vi "MessageHandler__LCR.vi"(6 "reference":T11, 7 "Data In":T3, 8 "error in (no error)":errorcluster, 9 "Action In":T4 caption="Action", 10 "Message":T1={"Command"=enum."SetPicture", "Parameter"=variant} caption="Messages", 11 "State In":T5={"Orientation"=0, "ActivePicture"={"image type"=0, "image depth"=0, "image"=[], "mask"=[], "colors"=[], "Rectangle"={"left"=0, "top"=0, "right"=0, "bottom"=0}}, "Pictures"={"Normal"={"image type"=0, "image depth"=0, "image"=[], "mask"=[], "colors"=[], "Rectangle"={"left"=0, "top"=0, "right"=0, "bottom"=0}}, "Hilite"={"image type"=0, "image depth"=0, "image"=[], "mask"=[], "colors"=[], "Rectangle"={"left"=0, "top"=0, "right"=0, "bottom"=0}}}, "Text"={"String"="", "Font"={"Font Name:"="", "Size"=0, "Strikeout?"=FALSE, "Italic?"=FALSE, "Underline?"=FALSE, "Outline?"=FALSE, "Shadow?"=FALSE, "Bold?"=FALSE}, "TextColor"=0}, "RunTimeSettings"={"Highlight"=FALSE, "ShowButton"=TRUE, "Behaviour"=enum."Switch when pressed", "React if disabled"=FALSE, "Nudge Button"=TRUE, "ShowButton on Hover"=FALSE, "Button Type"=enum."System"}, "Messages"=[], "Status"=0, "XControl Label"="", "Boolean Value"=FALSE} caption="State" {"Status" format="%.0x"}) -> (0 "error out":errorcluster, 1 "Action Out":T4 caption="Action", 2 "Remaining":i32, 3 "State Out":T5={"Orientation"=0, "ActivePicture"={"image type"=0, "image depth"=0, "image"=[], "mask"=[], "colors"=[], "Rectangle"={"left"=0, "top"=0, "right"=0, "bottom"=0}}, "Pictures"={"Normal"={"image type"=0, "image depth"=0, "image"=[], "mask"=[], "colors"=[], "Rectangle"={"left"=0, "top"=0, "right"=0, "bottom"=0}}, "Hilite"={"image type"=0, "image depth"=0, "image"=[], "mask"=[], "colors"=[], "Rectangle"={"left"=0, "top"=0, "right"=0, "bottom"=0}}}, "Text"={"String"="", "Font"={"Font Name:"="", "Size"=0, "Strikeout?"=FALSE, "Italic?"=FALSE, "Underline?"=FALSE, "Outline?"=FALSE, "Shadow?"=FALSE, "Bold?"=FALSE}, "TextColor"=0}, "RunTimeSettings"={"Highlight"=FALSE, "ShowButton"=TRUE, "Behaviour"=enum."Switch when pressed", "React if disabled"=FALSE, "Nudge Button"=TRUE, "ShowButton on Hover"=FALSE, "Button Type"=enum."System"}, "Messages"=[], "Status"=0, "XControl Label"="", "Boolean Value"=FALSE} caption="State" {"Status" format="%.0x"})   [LabVIEW 2011, in "BooleanXControl__LCR.xctl"]
uses:
  BooleanXControl__LCR.xctl
  Controls/BX.Refs__LCR.ctl
  Abilities/BX.State__LCR.ctl
  Controls/BX.Orientation__LCR.ctl
  <vilib>/picture/picture.llb/imagedata.ctl
  Controls/BX.RTSettings__LCR.ctl
  Controls/BX.Behaviour__LCR.ctl
  Controls/BX.ButtonType__LCR.ctl
  Controls/BX.Message__LCR.ctl
  Controls/BX.Commands__LCR.ctl
  <vilib>/_xctls/Action.ctl
  Abilities/BX.Data__LCR.ctl
  <vilib>/_xctls/XControlSupport.lvlib
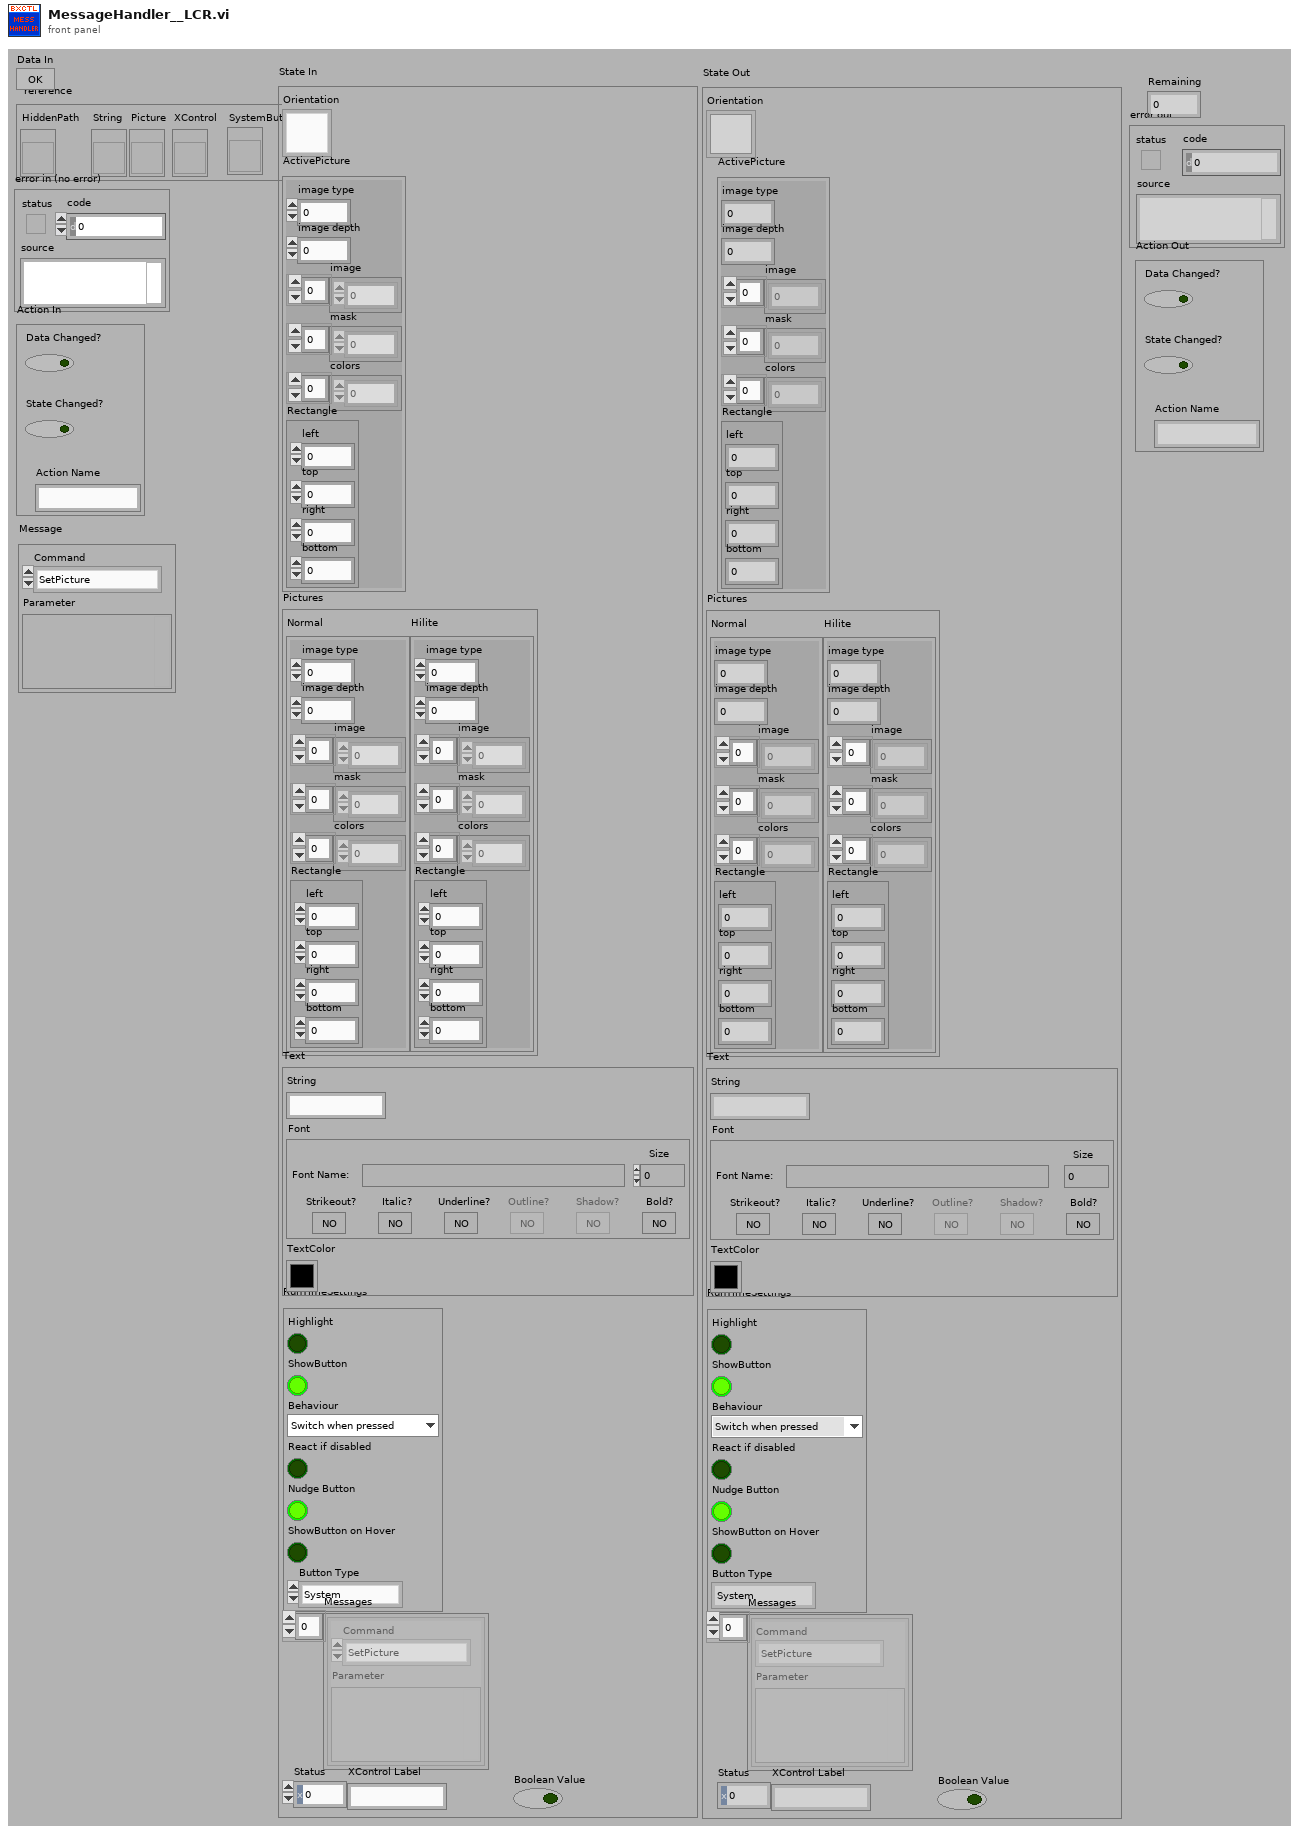
[diagram p1: front panel]
types:
  T1 = typedef "BooleanXControl__LCR.xctl/BX.Message__LCR.ctl" = cluster{"Command":T2, "Parameter":variant}
  T2 = typedef "BooleanXControl__LCR.xctl/BX.Commands__LCR.ctl" = enum16{"None", "SetPicture", "SetFont", "SetText", "SetOrientation", "Redraw", "SetTextColor", "SetRTSettings", "MultipleUpdate", "RT.Button", "RT.Hilite", "RT.Behaviour", "RT.Disabled", "ShowGUI", "RT.Nudge", "RT.Hover", "RT.ButtonType"}
  T3 = typedef "BooleanXControl__LCR.xctl/BX.Data__LCR.ctl" = bool
  T4 = typedef "XControlSupport.lvlib/Action.ctl" = cluster{"Data Changed?":bool, "State Changed?":bool, "Action Name":string}
  T5 = typedef "BooleanXControl__LCR.xctl/BX.State__LCR.ctl" = cluster{"Orientation":T6, "ActivePicture":T7, "Pictures":cluster{"Normal":T7, "Hilite":T7}, "Text":cluster{"String":string, "Font":cluster{"Font Name:":string, "Size":i16, "Strikeout?":bool, "Italic?":bool, "Underline?":bool, "Outline?":bool, "Shadow?":bool, "Bold?":bool}, "TextColor":u32}, "RunTimeSettings":T8, "Messages":T1[], "Status":u16, "XControl Label":string, "Boolean Value":bool}
  T6 = typedef "BooleanXControl__LCR.xctl/BX.Orientation__LCR.ctl" = u8
  T7 = typedef "imagedata.ctl" = cluster{"image type":i32, "image depth":i32, "image":u8[], "mask":u8[], "colors":u32[], "Rectangle":cluster{"left":i16, "top":i16, "right":i16, "bottom":i16}}
  T8 = typedef "BooleanXControl__LCR.xctl/BX.RTSettings__LCR.ctl" = cluster{"Highlight":bool, "ShowButton":bool, "Behaviour":T9, "React if disabled":bool, "Nudge Button":bool, "ShowButton on Hover":bool, "Button Type":T10}
  T9 = typedef "BooleanXControl__LCR.xctl/BX.Behaviour__LCR.ctl" = enum16{"Switch when pressed", "Switch when released", "Switch until released"}
  T10 = typedef "BooleanXControl__LCR.xctl/BX.ButtonType__LCR.ctl" = enum16{"System", "Modern", "Classic", "Decoration"}
  T11 = typedef "BooleanXControl__LCR.xctl/BX.Refs__LCR.ctl" = cluster{"HiddenPath":refnum<vi>, "String":refnum<vi>, "Picture":refnum<vi>, "XControl":refnum<vi>, "SystemButton":refnum<vi>, "ModernButton":refnum<vi>, "ClassicButton":refnum<vi>, "Decor Refnum":refnum<vi>}
  T12 = cluster{"Font Name:":string, "Size":i16, "Strikeout?":bool, "Italic?":bool, "Underline?":bool, "Outline?":bool, "Shadow?":bool, "Bold?":bool}
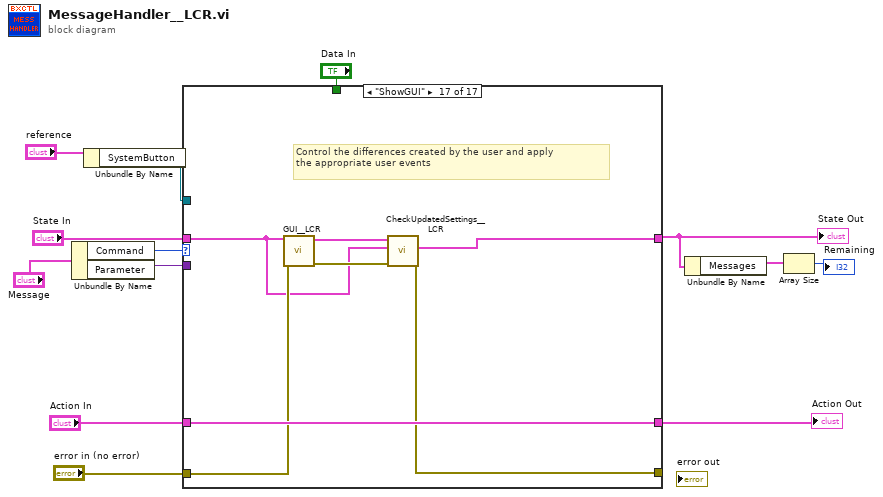
[diagram p0: block diagram]
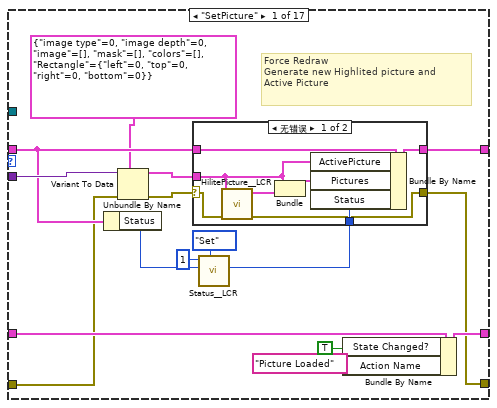
[diagram p2: hidden frame]
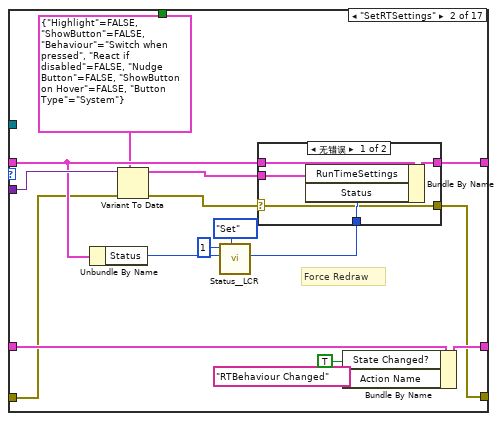
[diagram p4: hidden frame]
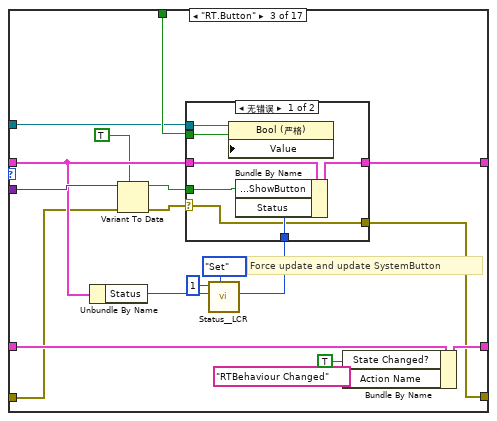
[diagram p6: hidden frame]
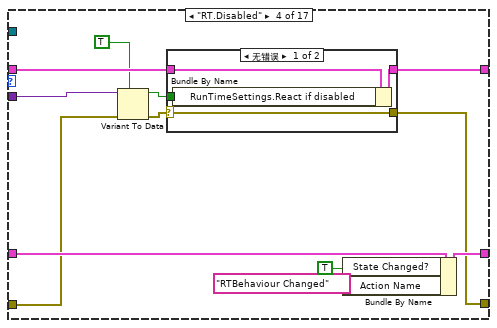
[diagram p8: hidden frame]
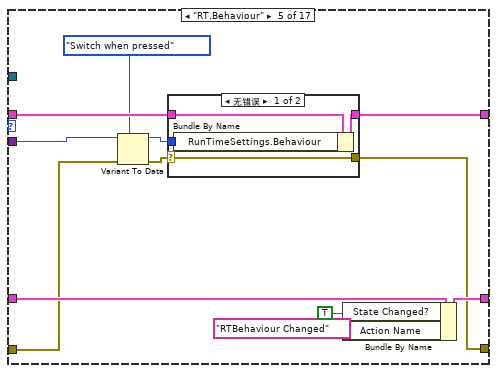
[diagram p10: hidden frame]
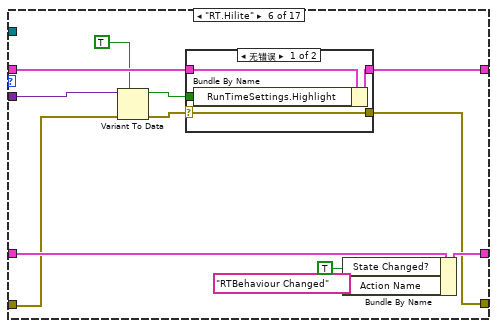
[diagram p12: hidden frame]
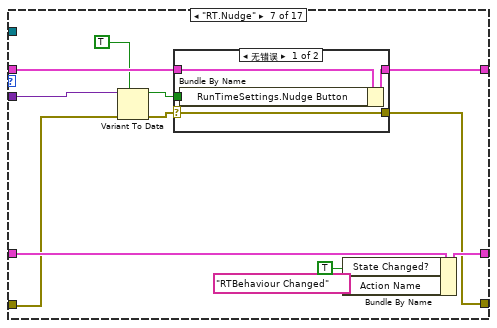
[diagram p14: hidden frame]
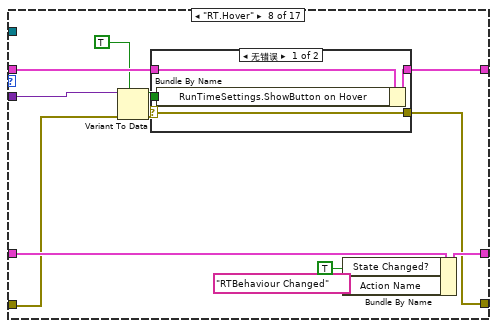
[diagram p16: hidden frame]
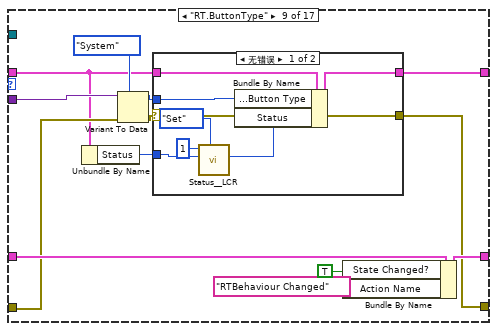
[diagram p18: hidden frame]
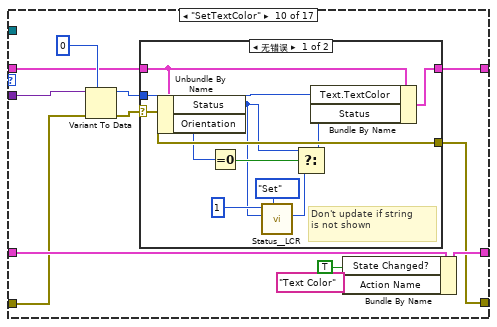
[diagram p20: hidden frame]
diagram:
  n1 = Unbundle By Name("Message") -> ("Command"=w5:T2, "Parameter"=w4:variant)
  n2 = Unbundle By Name("reference") -> ("SystemButton"=w8:refnum<vi>)
  n3 = case shown="\"ShowGUI\"" w5 {
    tunnel: w4 -> [w28 w54 w79 w100 w118 w136 w154 w172 w191 w213 w239 w264 w288 _ _ w322 _]
    tunnel: "State In" -> [w22 w48 w73 w94 w112 w130 w148 w166 w181 w206 w229 w255 w281 w309 w313 w315 w328]
    tunnel: "Action In" -> [w27 w53 w78 w99 w117 w135 w153 w171 w190 w211 w238 w263 w287 w310 w312 w323 w333]
    tunnel: [w26 w52 w77 w98 w116 w134 w152 w170 w189 w210 w237 w262 w286 w310 w312 w323 w333] -> w12
    tunnel: [w29 w55 w80 w101 w119 w137 w155 w173 w192 w214 w228 w254 w289 w308 w313 w314 w329] -> w3
    tunnel: "error in (no error)" -> [w19 w45 w70 w91 w109 w127 w145 w163 w183 w204 w233 w258 w279 w307 w311 w318 w332]
    tunnel: [w18 w44 w69 w90 w108 w126 w144 w162 w182 w203 w232 w253 w278 w307 w311 w316 w330] -> _
    tunnel: "Data In" -> [_ _ w68 _ _ _ _ _ _ _ _ _ _ _ _ _ _]
    tunnel: w8 -> [_ _ w67 _ _ _ _ _ _ _ _ _ _ _ _ _ _]
    frame "SetPicture" {
      # "Force Redraw\nGenerate new Highlited picture and\nActive Picture"
      n4 = Unbundle By Name(w22) -> ("Status"=w17:u16)
      n5 = Variant To Data(error in=w19, type=T7 {"image type"=0, "image depth"=0, "image"=[], "mask"=[], "colors"=[], "Rectangle"={"left"=0, "top"=0, "right"=0, "bottom"=0}} ("image data"), Variant=w28) -> (data=w23:T7, error out=w21:errorcluster)
      n6 = call "Status__LCR.vi"("Action (Get)"=enum16{"Get", "Set", "Reset"}."Set", "Status In"=w17, "Bit"=u16 1) -> ("Status Out"=w14:u16)  [unwired: 7 in, 1 out]
      n7 = case shown="无错误" w21 {
        selector: w21 -> [w31 w38]
        tunnel: [w37 w39] -> w29
        tunnel: w23 -> [w34 _]
        tunnel: w22 -> [w33 w39]
        tunnel: w14 -> [w32 _]
        tunnel: [w30 w38] -> w18
        frame No Error {
          n8 = call "HilitePicture__LCR.vi"("error in (no error)"=w31, "image data"=w34) -> ("error out"=w30:errorcluster, "Hilited Picture"=w36:T7)  [unwired: 8 in]
          n9 = Bundle("image data"=w34, "Hilited Picture"=w36) -> (w35:cluster{"image data":T7, "Hilited Picture":T7})  [unwired: 1 in]
          n10 = Bundle By Name(cluster=w33, "ActivePicture"=w34, "Pictures"=w35, "Status"=w32) -> (w37:T5)
        }
        frame Error {
          # "Wrong datatype"
        }
      }
      n11 = Bundle By Name(cluster=w27, "State Changed?"=TRUE ("Data Changed?"), "Action Name"="Picture Loaded") -> (w26:T4)
    }
    frame "SetRTSettings" {
      # "Force Redraw"
      n12 = Unbundle By Name(w48) -> ("Status"=w41:u16)
      n13 = Variant To Data(error in=w45, type=T8 {"Highlight"=FALSE, "ShowButton"=FALSE, "Behaviour"=enum."Switch when pressed", "React if disabled"=FALSE, "Nudge Button"=FALSE, "ShowButton on Hover"=FALSE, "Button Type"=enum."System"} ("RunTimeSettings"), Variant=w54) -> (data=w49:T8, error out=w47:errorcluster)
      n14 = call "Status__LCR.vi"("Action (Get)"=enum16{"Get", "Set", "Reset"}."Set", "Status In"=w41, "Bit"=u16 1) -> ("Status Out"=w40:u16)  [unwired: 7 in, 1 out]
      n15 = case shown="无错误" w47 {
        selector: w47 -> [w56 w61]
        tunnel: [w60 w62] -> w55
        tunnel: w49 -> [w59 _]
        tunnel: w48 -> [w58 w62]
        tunnel: w40 -> [w57 _]
        tunnel: [w56 w61] -> w44
        frame No Error {
          n16 = Bundle By Name(cluster=w58, "RunTimeSettings"=w59, "Status"=w57) -> (w60:T5)
        }
        frame Error {
          # "Wrong Datatype"
        }
      }
      n17 = Bundle By Name(cluster=w53, "State Changed?"=TRUE ("Data Changed?"), "Action Name"="RTBehaviour Changed") -> (w52:T4)
    }
    frame "RT.Button" {
      # "Force update and update SystemButton"
      n18 = Unbundle By Name(w73) -> ("Status"=w64:u16)
      n19 = Variant To Data(error in=w70, type=TRUE, Variant=w79) -> (data=w74:bool, error out=w72:errorcluster)
      n20 = call "Status__LCR.vi"("Action (Get)"=enum16{"Get", "Set", "Reset"}."Set", "Status In"=w64, "Bit"=u16 1) -> ("Status Out"=w63:u16)  [unwired: 7 in, 1 out]
      n21 = case shown="无错误" w72 {
        selector: w72 -> [w83 w88]
        tunnel: [w87 w89] -> w80
        tunnel: w74 -> [w86 _]
        tunnel: w73 -> [w85 w89]
        tunnel: w63 -> [w84 _]
        tunnel: [w83 w88] -> w69
        tunnel: w68 -> [w82 _]
        tunnel: w67 -> [w81 _]
        frame No Error {
          n22 = property class="Bool (严格)"(reference=w81, "Value"=w82) -> ()  [unwired: 1 in, 2 out]
          n23 = Bundle By Name(cluster=w85, "RunTimeSettings.ShowButton"=w86, "Status"=w84) -> (w87:T5)
        }
        frame Error {
          # "Wrong datatype"
        }
      }
      n24 = Bundle By Name(cluster=w78, "State Changed?"=TRUE ("Data Changed?"), "Action Name"="RTBehaviour Changed") -> (w77:T4)
    }
    frame "RT.Disabled" {
      n25 = Variant To Data(error in=w91, type=TRUE, Variant=w100) -> (data=w95:bool, error out=w93:errorcluster)
      n26 = case shown="无错误" w93 {
        selector: w93 -> [w102 w106]
        tunnel: [w105 w107] -> w101
        tunnel: w95 -> [w104 _]
        tunnel: w94 -> [w103 w107]
        tunnel: [w102 w106] -> w90
        frame No Error {
          n27 = Bundle By Name(cluster=w103, "RunTimeSettings.React if disabled"=w104) -> (w105:T5)
        }
        frame Error {
          # "Wrong Datatype"
        }
      }
      n28 = Bundle By Name(cluster=w99, "State Changed?"=TRUE ("Data Changed?"), "Action Name"="RTBehaviour Changed") -> (w98:T4)
    }
    frame "RT.Behaviour" {
      n29 = Variant To Data(error in=w109, type=BX.Behaviour__LCR."Switch when pressed" ("Behaviour"), Variant=w118) -> (data=w113:T9, error out=w111:errorcluster)
      n30 = case shown="无错误" w111 {
        selector: w111 -> [w120 w124]
        tunnel: [w123 w125] -> w119
        tunnel: w113 -> [w122 _]
        tunnel: w112 -> [w121 w125]
        tunnel: [w120 w124] -> w108
        frame No Error {
          n31 = Bundle By Name(cluster=w121, "RunTimeSettings.Behaviour"=w122) -> (w123:T5)
        }
        frame Error {
          # "Wrong Datatype"
        }
      }
      n32 = Bundle By Name(cluster=w117, "State Changed?"=TRUE ("Data Changed?"), "Action Name"="RTBehaviour Changed") -> (w116:T4)
    }
    frame "RT.Hilite" {
      n33 = Variant To Data(error in=w127, type=TRUE, Variant=w136) -> (data=w131:bool, error out=w129:errorcluster)
      n34 = case shown="无错误" w129 {
        selector: w129 -> [w138 w142]
        tunnel: [w141 w143] -> w137
        tunnel: w131 -> [w140 _]
        tunnel: w130 -> [w139 w143]
        tunnel: [w138 w142] -> w126
        frame No Error {
          n35 = Bundle By Name(cluster=w139, "RunTimeSettings.Highlight"=w140) -> (w141:T5)
        }
        frame Error {
          # "Wrong Datatype"
        }
      }
      n36 = Bundle By Name(cluster=w135, "State Changed?"=TRUE ("Data Changed?"), "Action Name"="RTBehaviour Changed") -> (w134:T4)
    }
    frame "RT.Nudge" {
      n37 = Variant To Data(error in=w145, type=TRUE, Variant=w154) -> (data=w149:bool, error out=w147:errorcluster)
      n38 = case shown="无错误" w147 {
        selector: w147 -> [w156 w160]
        tunnel: [w159 w161] -> w155
        tunnel: w149 -> [w158 _]
        tunnel: w148 -> [w157 w161]
        tunnel: [w156 w160] -> w144
        frame No Error {
          n39 = Bundle By Name(cluster=w157, "RunTimeSettings.Nudge Button"=w158) -> (w159:T5)
        }
        frame Error {
          # "Wrong Datatype"
        }
      }
      n40 = Bundle By Name(cluster=w153, "State Changed?"=TRUE ("Data Changed?"), "Action Name"="RTBehaviour Changed") -> (w152:T4)
    }
    frame "RT.Hover" {
      n41 = Variant To Data(error in=w163, type=TRUE, Variant=w172) -> (data=w167:bool, error out=w165:errorcluster)
      n42 = case shown="无错误" w165 {
        selector: w165 -> [w174 w178]
        tunnel: [w177 w179] -> w173
        tunnel: w167 -> [w176 _]
        tunnel: w166 -> [w175 w179]
        tunnel: [w174 w178] -> w162
        frame No Error {
          n43 = Bundle By Name(cluster=w175, "RunTimeSettings.ShowButton on Hover"=w176) -> (w177:T5)
        }
        frame Error {
          # "Wrong Datatype"
        }
      }
      n44 = Bundle By Name(cluster=w171, "State Changed?"=TRUE ("Data Changed?"), "Action Name"="RTBehaviour Changed") -> (w170:T4)
    }
    frame "RT.ButtonType" {
      n45 = Unbundle By Name(w181) -> ("Status"=w180:u16)
      n46 = Variant To Data(error in=w183, type=BX.ButtonType__LCR."System", Variant=w191) -> (data=w186:T10, error out=w185:errorcluster)
      n47 = case shown="无错误" w185 {
        selector: w185 -> [w197 w201]
        tunnel: [w200 w202] -> w192
        tunnel: w186 -> [w199 _]
        tunnel: w181 -> [w198 w202]
        tunnel: [w197 w201] -> w182
        tunnel: w180 -> [w196 _]
        frame No Error {
          n48 = call "Status__LCR.vi"("Action (Get)"=enum16{"Get", "Set", "Reset"}."Set", "Status In"=w196, "Bit"=u16 1) -> ("Status Out"=w193:u16)  [unwired: 7 in, 1 out]
          n49 = Bundle By Name(cluster=w198, "RunTimeSettings.Button Type"=w199, "Status"=w193) -> (w200:T5)
        }
        frame Error {
          # "Wrong Datatype"
        }
      }
      n50 = Bundle By Name(cluster=w190, "State Changed?"=TRUE ("Data Changed?"), "Action Name"="RTBehaviour Changed") -> (w189:T4)
    }
    frame "SetTextColor" {
      n51 = Variant To Data(error in=w204, type=u32 0, Variant=w213) -> (data=w212:u32, error out=w205:errorcluster)
      n52 = case shown="无错误" w205 {
        selector: w205 -> [w222 w226]
        tunnel: [w225 w227] -> w214
        tunnel: w212 -> [w224 _]
        tunnel: w206 -> [w223 w227]
        tunnel: [w222 w226] -> w203
        frame No Error {
          # "Don't update if string\nis not shown"
          n53 = Unbundle By Name(w223) -> ("Status"=w216:u16, "Orientation"=w221:T6)
          n54 = Equal To 0?(x=w221) -> (x = 0?=w220:bool)
          n55 = call "Status__LCR.vi"("Action (Get)"=enum16{"Get", "Set", "Reset"}."Set", "Status In"=w216, "Bit"=u16 1) -> ("Status Out"=w215:u16)  [unwired: 7 in, 1 out]
          n56 = Select(t=w216, s=w220, f=w215) -> (s? t:f=w217:u16)
          n57 = Bundle By Name(cluster=w223, "Text.TextColor"=w224, "Status"=w217) -> (w225:T5)
        }
        frame Error {
          # "Wrong datatype"
        }
      }
      n58 = Bundle By Name(cluster=w211, "State Changed?"=TRUE ("Data Changed?"), "Action Name"="Text Color") -> (w210:T4)
    }
    frame "SetFont" {
      n59 = Variant To Data(error in=w233, type=T12 {"Font Name:"="", "Size"=0, "Strikeout?"=FALSE, "Italic?"=FALSE, "Underline?"=FALSE, "Outline?"=FALSE, "Shadow?"=FALSE, "Bold?"=FALSE} ("user-specified font"), Variant=w239) -> (data=w230:T12, error out=w231:errorcluster)
      n60 = case shown="无错误" w231 {
        selector: w231 -> [w247 w251]
        tunnel: [w250 w252] -> w228
        tunnel: w230 -> [w249 _]
        tunnel: w229 -> [w248 w252]
        tunnel: [w247 w251] -> w232
        frame No Error {
          # "Don't update if string\nis not shown"
          n61 = Unbundle By Name(w248) -> ("Status"=w241:u16, "Orientation"=w246:T6)
          n62 = Equal To 0?(x=w246) -> (x = 0?=w245:bool)
          n63 = call "Status__LCR.vi"("Action (Get)"=enum16{"Get", "Set", "Reset"}."Set", "Status In"=w241, "Bit"=u16 1) -> ("Status Out"=w240:u16)  [unwired: 7 in, 1 out]
          n64 = Select(t=w241, s=w245, f=w240) -> (s? t:f=w242:u16)
          n65 = Bundle By Name(cluster=w248, "Text.Font"=w249, "Status"=w242) -> (w250:T5)
        }
        frame Error {
          # "Wrong datatype"
        }
      }
      n66 = Bundle By Name(cluster=w238, "State Changed?"=TRUE ("Data Changed?"), "Action Name"="Font Set") -> (w237:T4)
    }
    frame "SetText" {
      n67 = Variant To Data(error in=w258, type="", Variant=w264) -> (data=w257:string, error out=w256:errorcluster)
      n68 = case shown="无错误" w256 {
        selector: w256 -> [w272 w276]
        tunnel: [w275 w277] -> w254
        tunnel: w257 -> [w274 _]
        tunnel: w255 -> [w273 w277]
        tunnel: [w272 w276] -> w253
        frame No Error {
          # "Don't update if string\nis not shown"
          n69 = Unbundle By Name(w273) -> ("Status"=w266:u16, "Orientation"=w271:T6)
          n70 = Equal To 0?(x=w271) -> (x = 0?=w270:bool)
          n71 = call "Status__LCR.vi"("Action (Get)"=enum16{"Get", "Set", "Reset"}."Set", "Status In"=w266, "Bit"=u16 1) -> ("Status Out"=w265:u16)  [unwired: 7 in, 1 out]
          n72 = Select(t=w266, s=w270, f=w265) -> (s? t:f=w267:u16)
          n73 = Bundle By Name(cluster=w273, "Text.String"=w274, "Status"=w267) -> (w275:T5)
        }
        frame Error {
          # "Wrong datatype"
        }
      }
      n74 = Bundle By Name(cluster=w263, "State Changed?"=TRUE ("Data Changed?"), "Action Name"="Text Set") -> (w262:T4)
    }
    frame "SetOrientation" {
      n75 = Variant To Data(error in=w279, type=T6 0 ("Orientations"), Variant=w288) -> (data=w283:T6, error out=w280:errorcluster)
      n76 = case shown="无错误" w280 {
        selector: w280 -> [w298 w301]
        tunnel: [w300 w302] -> w289
        tunnel: w283 -> [w297 _]
        tunnel: w281 -> [w299 w302]
        tunnel: [w298 w301] -> w278
        frame No Error {
          # "Force Redraw if orientation changed"
          n77 = Unbundle By Name(w299) -> ("Status"=w292:u16, "Orientation"=w290:T6)
          n78 = Equal?(x=w290, y=w297) -> (x = y?=w293:bool)
          n79 = call "Status__LCR.vi"("Action (Get)"=enum16{"Get", "Set", "Reset"}."Set", "Status In"=w292, "Bit"=u16 1) -> ("Status Out"=w294:u16)  [unwired: 7 in, 1 out]
          n80 = Select(t=w292, s=w293, f=w294) -> (s? t:f=w291:u16)
          n81 = Bundle By Name(cluster=w299, "Orientation"=w297, "Status"=w291) -> (w300:T5)
        }
        frame Error {
          # "Wrong Datatype"
        }
      }
      n82 = Bundle By Name(cluster=w287, "State Changed?"=TRUE ("Data Changed?"), "Action Name"="Orientation Set") -> (w286:T4)
    }
    frame "Redraw" {
      # "Force Redraw"
      n83 = Unbundle By Name(w309) -> ("Status"=w303:u16)
      n84 = call "Status__LCR.vi"("Action (Get)"=enum16{"Get", "Set", "Reset"}."Set", "Status In"=w303, "Bit"=u16 1) -> ("Status Out"=w304:u16)  [unwired: 7 in, 1 out]
      n85 = Bundle By Name(cluster=w309, "Status"=w304) -> (w308:T5)
    }
    frame "None" {
      # "Bogus entry"
    }
    frame "MultipleUpdate" {
      # "Generate an event for every element"
      n86 = Variant To Data(error in=w318, type=T1[] [], Variant=w322) -> (data=w320:T1[], error out=w319:errorcluster)
      n87 = for {
        tunnel: w320 -> [w326] mode=indexing
        tunnel: w319 -> [w324]
        tunnel: [w324] -> w317 mode=indexing
        shift-right: [w325] -> w314
        shift-left: w315 -> [w327]
        n88 = call "AddMessageToState__LCR.vi"("Message"=w326, "State In"=w327) -> ("State Out"=w325:T5)  [unwired: 9 in]
      }
      n89 = Merge Errors(w317) -> (w316:errorcluster)
    }
    frame "ShowGUI" {
      # "Control the differences created by the user and apply\nthe appropriate user events"
      n90 = call "GUI__LCR.vi"("error in"=w332, "State In"=w328) -> ("error out"=w331:errorcluster, "State Out"=w334:T5)  [unwired: 8 in]
      n91 = call "CheckUpdatedSettings__LCR.vi"("error in (no error)"=w331, "Old State"=w328, "New State"=w334) -> ("error out"=w330:errorcluster, "State Out"=w329:T5)  [unwired: 7 in]
    }
  }
  "Action Out" <- w12
  "State Out" <- w3
  n92 = Unbundle By Name(w3) -> ("Messages"=w2:T1[])
  n93 = Array Size(array=w2) -> (size(s)=→"Remaining":i32)
